vi "Load WAV.vi"(8 "error in":errorcluster, 11 "File":path) -> (0 "error out":errorcluster, 3 "Chunk Pointer":u32 format="%.0x")   [LabVIEW 2015, in "LibSDL2_Mixer.lvlib"]
uses:
  LibSDL2_Mixer.lvlib
  LibSDL2 Wrapper/LibSDL2.lvlib
  LibSDL2 Wrapper/DLL/SDL2_mixer.dll
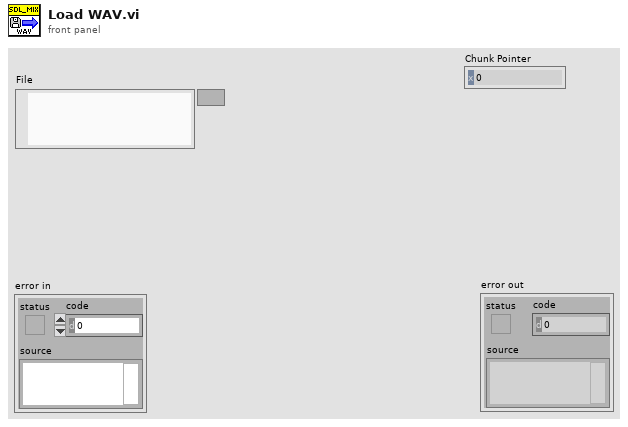
[diagram p1: front panel]
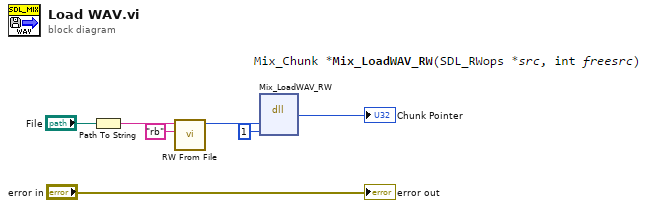
[diagram p0: block diagram]
diagram:
  n1 = Path To String(path="File") -> (string=w1:string)
  n2 = call "RW From File.vi"("Mode"="rb", "File"=w1) -> ("RWops Pointer"=w6:u32)  [unwired: 8 in, 1 out]
  n3 = dll-call lib="C:/dev/PGS/LabSDL2/Source/Libraries/LibSDL2 Wrapper/DLL/SDL2_mixer.dll" fn="Mix_LoadWAV_RW"("src"=w6, "freesrc"=1) -> ("return type"=→"Chunk Pointer":u32)  [unwired: 5 in, 2 out]
  "error out" <- "error in"
